vi "leer_LUZ.vi"() -> ()   [LabVIEW 2020]
uses:
  <vilib>/BLE/type_def/connection_status_bundle.ctl
  <vilib>/BLE/type_def/address_type.ctl
panel:
  out "Color":u32(colorbox)
  out "subarray":u8[](array[numeric])
  out "Connected 2":bool
  in  "Service UUID":string="EF6802009B3549339B1052FFA9740042"
  in  "Characteristic UUID":string="EF6802019B3549339B1052FFA9740042"
  out "Reading HR":bool
  in  "stop":bool
  out "Connected":bool
  in  "Address Type":T1=1 items=["Public", "Random"]
  out "Handle table":string[][](array[string])
  out "Connection Status":T2={"MAC Address"="", "cnx handle"=0, "cnx flags"=0, "Address Type"=125, "Connection Interval (ms)"=125, "Timeout(ms)"=125, "Latency"=0, "bonding handle"=0} {"Address Type" items=["Public", "Random"]}
  in  "Continue":bool
  in  "MAC Address":string
  in  "COM Bluegiga in":refnum<visa-resource-name>="COM13"
  out "BLED112 Dongle Info":string
  # "This VI an example of scanning for BLE devices using the \nBLED112 Bluetooth Smart Dongle by Bluegiga\nhttps://www.bluegiga.com/en-US/products/bled112-bluetooth-smart-dongle/\nand\nBLE  toolkit for LabVIEW\n\nInstructions:\nBefore running the VI\n1. Select the COM port for the BLED112 USB receiver\n(You can verify this in the Device Manager)\n\n2. Run the VI\n\n3. The VI will reset the dongle and scan for available BLE devices\n \n4. Introduce the MAC Address and Address Type of the HR monitor to connect and click in the CONTINUE button to connect with it\n\nYour device MUST compy with the BLE Heart Rate Profile\nhttps://developer.bluetooth.org/TechnologyOverview/Pages/HRP.aspx\n\n5. The VI will read the Characteristic 0x2A00 of the Service 0x1800 which contains \nthe Device Name\n\nhttps://www.bluetooth.com/specifications/gatt/viewer?attributeXmlFile=org.bluetooth.service.generic_access.xml&u=org.bluetooth.service.generic_access.xml\n\n6. Hear rate value will be updated\n\n7. Click in STOP to end the Hear Rate acqusition"
  # "SCAN"
  # "RSSI (power)"
  # "Advertising Package Type"
  # "MAC Address"
  # "Address Type"
  # "Friendly name"
  # "DEVICES FOUND"
  # "Introduce the MAC Address and Address Type of the device you want to connect and click in the CONTINUE button"
  # "CONNECT"
  # "READING DATA FROM DEVICE"
  # "Service 0x180D\nCharacteristic 0x2A37\nHeart Rate Measurement"
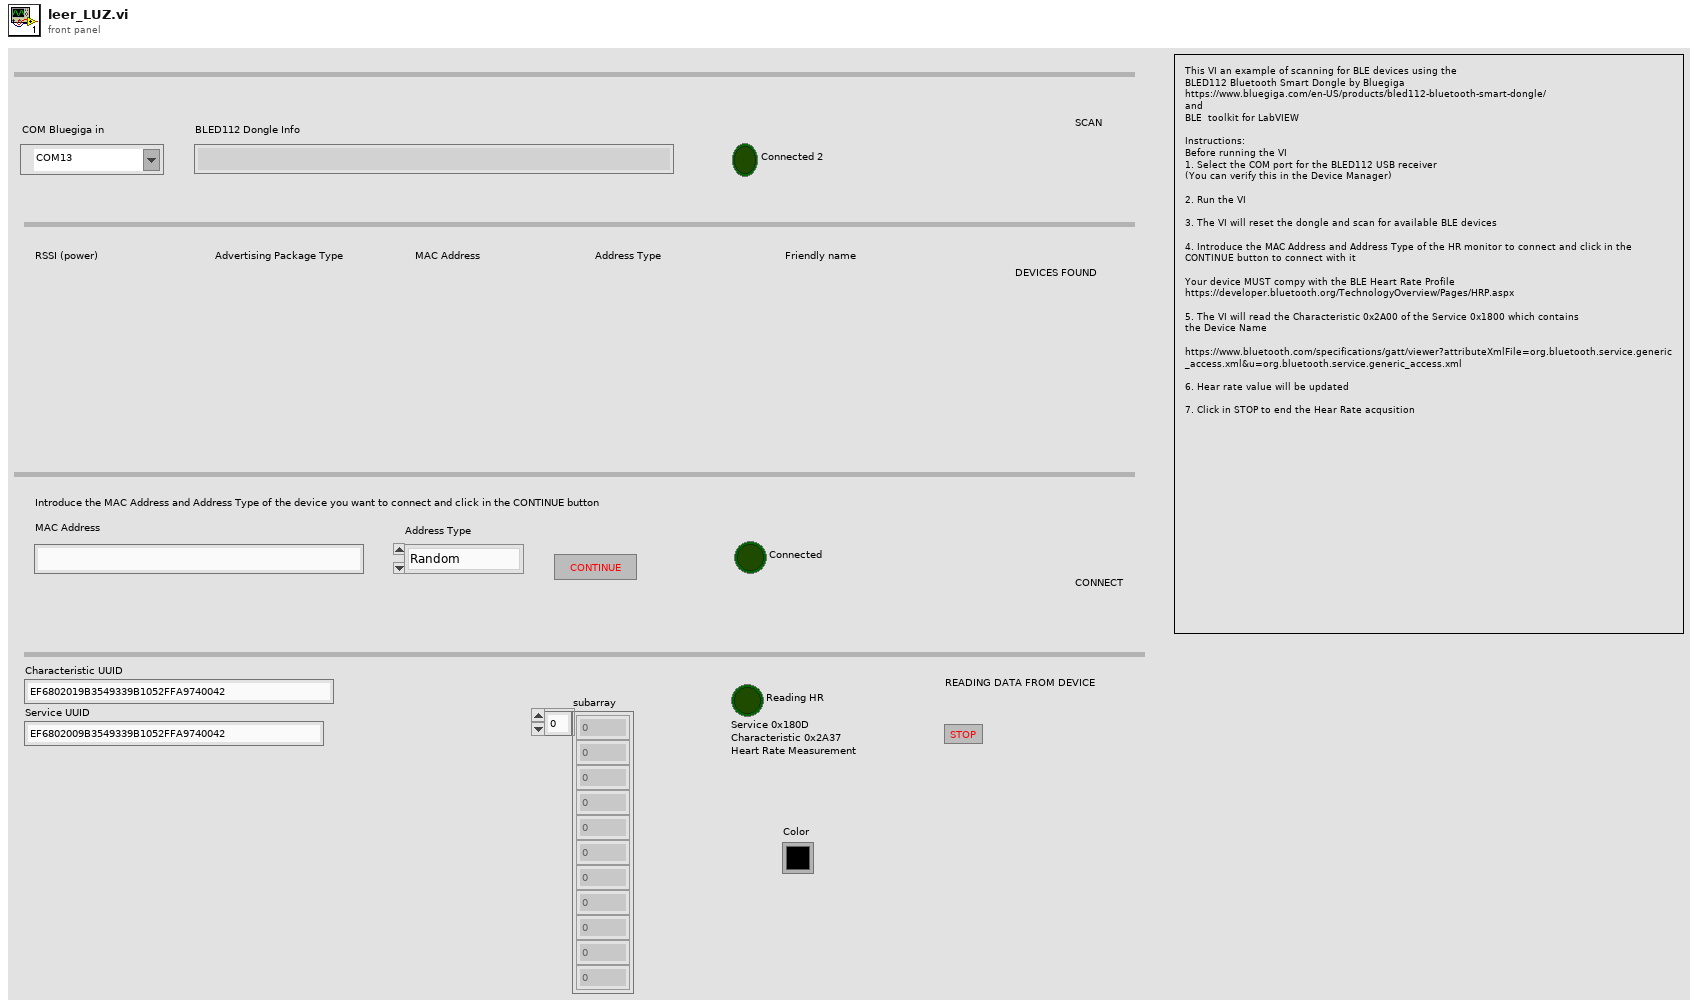
[diagram p1: front panel]
types:
  T1 = typedef "address_type.ctl" = u8
  T2 = typedef "connection_status_bundle.ctl" = cluster{"MAC Address":string, "cnx handle":u8, "cnx flags":u8, "Address Type":T1, "Connection Interval (ms)":u16, "Timeout(ms)":u16, "Latency":u16, "bonding handle":u8}
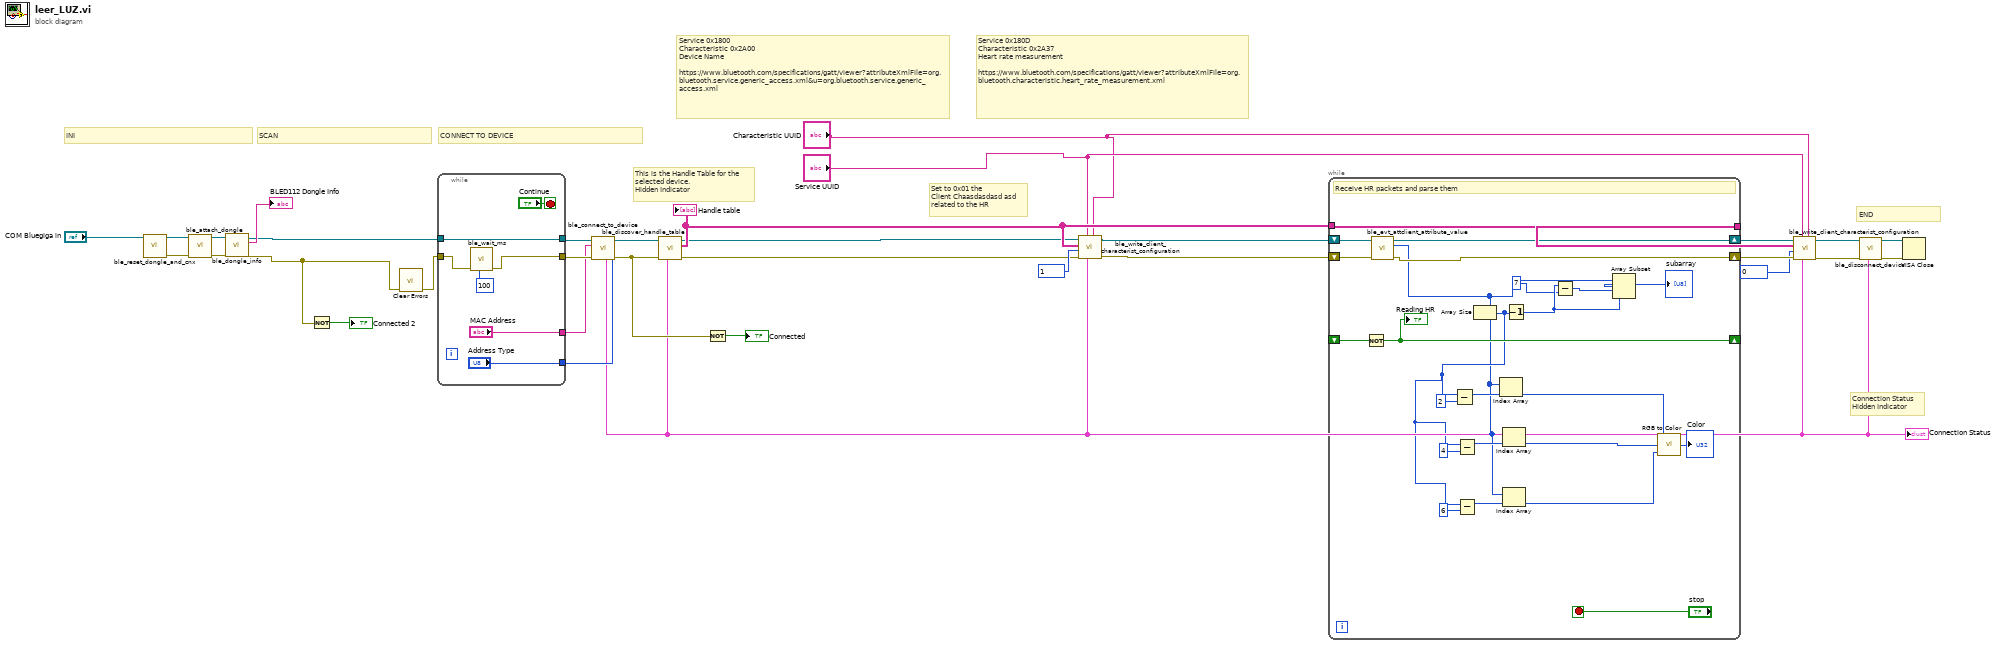
[diagram p0: block diagram]
diagram:
  # "Service 0x180D\nCharacteristic 0x2A37\nHeart rate measurement\n\nhttps://www.bluetooth.com/specifications/gatt/viewer?attributeXmlFile=org.bluetooth.characteristic.heart_rate_measurement.xml"
  # "Set to 0x01 the \nClient Chaasdasdasd asd\nrelated to the HR"
  # "Connection Status\nHidden Indicator"
  # "Service 0x1800\nCharacteristic 0x2A00\nDevice Name\n\nhttps://www.bluetooth.com/specifications/gatt/viewer?attributeXmlFile=org.bluetooth.service.generic_access.xml&u=org.bluetooth.service.generic_access.xml"
  # "This is the Handle Table for the\nselected device. \nHidden Indicator"
  # "CONNECT TO DEVICE"
  # "SCAN"
  # "END"
  # "INI"
  n1 = call <vilib>:"ble_reset_dongle_and_cnx.vi"("COM Bluegiga in"="COM Bluegiga in") -> ("error out"=w26:errorcluster, "COM Bluegiga out"=w24:refnum<visa-resource-name>)  [unwired: 9 in]
  n2 = call <vilib>:"ble_attach_dongle.vi"("error in (no error)"=w26, "COM Bluegiga in"=w24) -> ("error out"=w28:errorcluster, "COM Bluegiga out"=w27:refnum<visa-resource-name>)  [unwired: 8 in]
  n3 = call <vilib>:"ble_dongle_info.vi"("error in (no error)"=w28, "COM Bluegiga in"=w27) -> ("error out"=w2:errorcluster, "info"=→"BLED112 Dongle Info":string, "COM Bluegiga out"=w5:refnum<visa-resource-name>)  [unwired: 7 in]
  n4 = Not(x=w2) -> (.not. x?=→"Connected 2":bool)
  n5 = call <vilib>:"Clear Errors.vi"("error in (no error)"=w2) -> ("error out"=w22:errorcluster)  [unwired: 5 in, 1 out]
  n6 = while {
    tunnel: w22 -> [w40]
    tunnel: [w39] -> w33
    tunnel: w5 -> [w39]
    tunnel: [w38] -> w32
    tunnel: ["MAC Address"] -> w29
    tunnel: ["Address Type"] -> w21
    stop <- "Continue" stop-if-true
    n7 = call <vilib>:"ble_wait_ms.vi"("milliseconds to wait (100)"=u32 100, "error in (no error)"=w40) -> ("error out"=w38:errorcluster)  [unwired: 9 in]
  }
  n8 = call <vilib>:"ble_connect_to_device.vi"("Address Type"=w21, "error in (no error)"=w32, "MAC Address"=w29, "COM Bluegiga in"=w33) -> ("error out"=w19:errorcluster, "COM Bluegiga out"=w23:refnum<visa-resource-name>, "Connection Status"=w13:T2)  [unwired: 5 in]
  "Connection Status" <- w13
  n9 = call <vilib>:"ble_discover_handle_table.vi"("Connection Status"=w13, "error in (no error)"=w19, "COM Bluegiga in"=w23) -> ("error out"=w8:errorcluster, "Handle table"=w10:string[][], "COM Bluegiga out"=w9:refnum<visa-resource-name>)  [unwired: 6 in]
  "Handle table" <- w10
  n10 = Not(x=w19) -> (.not. x?=→"Connected":bool)
  n11 = call <vilib>:"ble_write_client_characterist_configuration.vi"("Characteristic UUID"="Characteristic UUID", "Connection Status"=w13, "Service UUID"="Service UUID", "error in (no error)"=w8, "Value(16bit)"=u16 1, "Handle table"=w10, "COM Bluegiga in"=w9) -> ("error out"=w6:errorcluster, "COM Bluegiga out"=w7:refnum<visa-resource-name>)  [unwired: 3 in]
  n12 = while {
    tunnel: w10 -> [w59]
    shift-right: [w62] -> w17
    shift-left: w7 -> [w65]
    shift-right: [w58] -> w18
    shift-left: w6 -> [w63]
    tunnel: [w59] -> w16
    shift-right: [w61] -> _
    shift-left: _ -> [w60]
    stop <- "stop" stop-if-true
    # "Receive HR packets and parse them"
    n13 = Not(x=w60) -> (.not. x?=w61:bool)
    "Reading HR" <- w61
    n14 = call <vilib>:"ble_evt_attclient_attribute_value.vi"("error in (no error)"=w63, "COM Bluegiga in"=w65) -> ("error out"=w58:errorcluster, "characteristic value"=w45:u8[], "COM Bluegiga out"=w62:refnum<visa-resource-name>)  [unwired: 6 in, 1 out]
    n15 = Array Size(array=w45) -> (size(s)=w46:i32)
    n16 = Subtract(x=w46, y=2) -> (x-y=w52:i32)
    n17 = Subtract(x=w46, y=4) -> (x-y=w50:i32)
    n18 = Subtract(x=w46, y=6) -> (x-y=w48:i32)
    n19 = Index Array(array=w45, index=w52) -> (element=w53:u8)
    n20 = Index Array(array=w45, index=w50) -> (element=w44:u8)
    n21 = Index Array(array=w45, index=w48) -> (element=w43:u8)
    n22 = Decrement(x=w46) -> (x-1=w55:i32)
    n23 = Subtract(x=w55, y=7 ("x")) -> (x-y=w56:i32)
    n24 = Array Subset(array=w45, index=w56, length=w55) -> (→"subarray":u8[])
    n25 = call <vilib>:"RGB to Color.vi"("B"=w43, "G"=w44, "R"=w53) -> ("Color"=→"Color":u32)
  }
  n26 = call <vilib>:"ble_write_client_characterist_configuration.vi"("Characteristic UUID"="Characteristic UUID", "Connection Status"=w13, "Service UUID"="Service UUID", "error in (no error)"=w18, "Value(16bit)"=u16 0, "Handle table"=w16, "COM Bluegiga in"=w17) -> ("error out"=w14:errorcluster, "COM Bluegiga out"=w15:refnum<visa-resource-name>)  [unwired: 3 in]
  n27 = call <vilib>:"ble_disconnect_device.vi"("Connection Status"=w13, "error in (no error)"=w14, "COM Bluegiga in"=w15) -> ("error out"=w30:errorcluster, "COM Bluegiga out"=w31:refnum<visa-resource-name>)  [unwired: 7 in]
  n28 = VISA Close(VISA resource name=w31, error in (no error)=w30) -> ()  [unwired: 1 out]
